vi "ConfigureSequencer.vi"(3 "error in (no error)":errorcluster, 4 "Sequencer":T1(array[cluster])=[{"Entry Length"=16384, "Repetition Count"=1, "Infinite Repetitions"=FALSE, "Channels"=[{"Analog Waveform"="SINE", "Amplitude [V]"=0.0, "Offset [V]"=0.0}, {"Analog Waveform"="SINE", "Amplitude [V]"=0.0, "Offset [V]"=0.0}], "Digital Waveform"=""}] {"Repetition Count" min=1}, 5 "VISA resource name":refnum<visa-resource-name>) -> (0 "error out":errorcluster, 2 "VISA resource name out":refnum<visa-resource-name>)   [LabVIEW 2020, in "Active Technologies AWG3000.lvlib"]
uses:
  Active Technologies AWG3000.lvlib
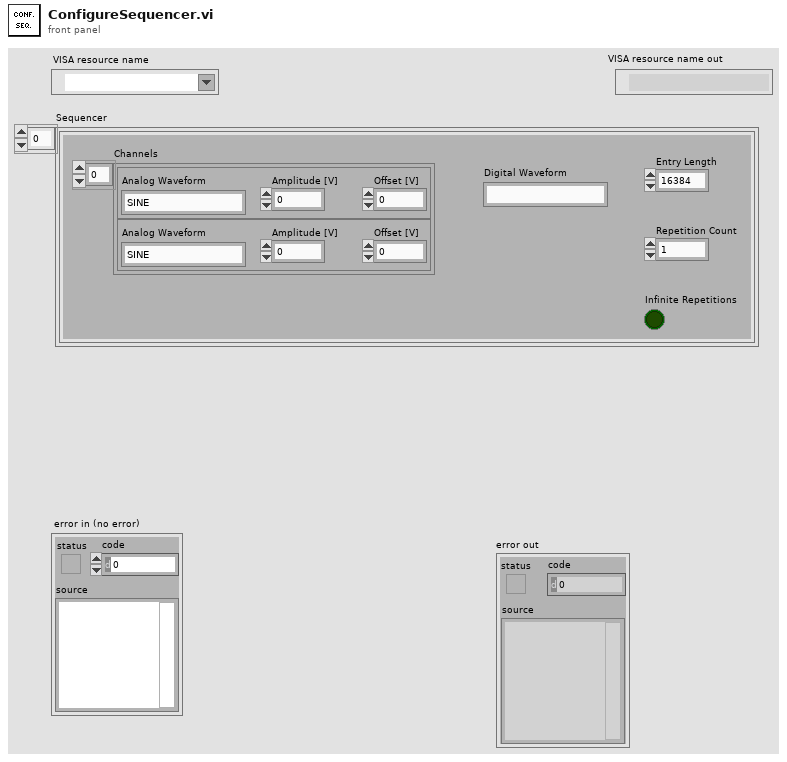
[diagram p1: front panel]
types:
  T1 = cluster{"Entry Length":i32, "Repetition Count":i32, "Infinite Repetitions":bool, "Channels":cluster{"Analog Waveform":string, "Amplitude [V]":dbl, "Offset [V]":dbl}[], "Digital Waveform":string}[]
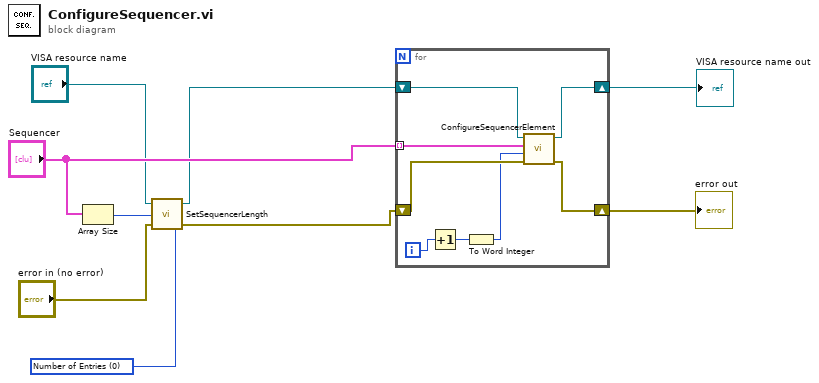
[diagram p0: block diagram]
diagram:
  w3 = u16 0 items=["Number of Entries", "Default", "Minimum", "Maximum"] ("Sequencer Length Options")
  n1 = Array Size(array="Sequencer") -> (size(s)=w4:i32)
  n2 = call "SetSequencerLength.vi"("Sequencer Length Options"=w3, "error in (no error)"="error in (no error)", "Number of Entries"=w4, "VISA resource name"="VISA resource name") -> ("error out"=w1:errorcluster, "VISA resource name out"=w2:refnum<visa-resource-name>)
  n3 = for {
    shift-right: [w16] -> w9
    shift-left: w2 -> [w17]
    shift-right: [w14] -> w8
    shift-left: w1 -> [w15]
    tunnel: "Sequencer" -> [w13] mode=indexing
    i -> [w12]
    n4 = Increment(x=w12) -> (x+1=w11:i32)
    n5 = To Word Integer(number=w11) -> (16bit integer=w10:i16)
    n6 = call "ConfigureSequencerElement.vi"("error in (no error)"=w15, "Sequencer Element"=w10, "Sequencer Item"=w13, "VISA resource name"=w17) -> ("error out"=w14:errorcluster, "VISA resource name out"=w16:refnum<visa-resource-name>)  [unwired: 2 in]
  }
  "VISA resource name out" <- w9
  "error out" <- w8
